vi "BusB FINS initialization Packet Encode.vi"(8 "error in":errorcluster, 11 "BusB Initialization Parameters":T1) -> (0 "error out":errorcluster, 2 "FCC Navigation send byte Array":u8[](array[numeric]) format="%x", 3 "BusB Initialization Parameters out":T1)   [LabVIEW 2016, in "Impedance Data Acquisition and Decoding.lvlib"]
uses:
  Impedance Data Acquisition and Decoding.lvlib
  BusB Initialization Parameters.ctl
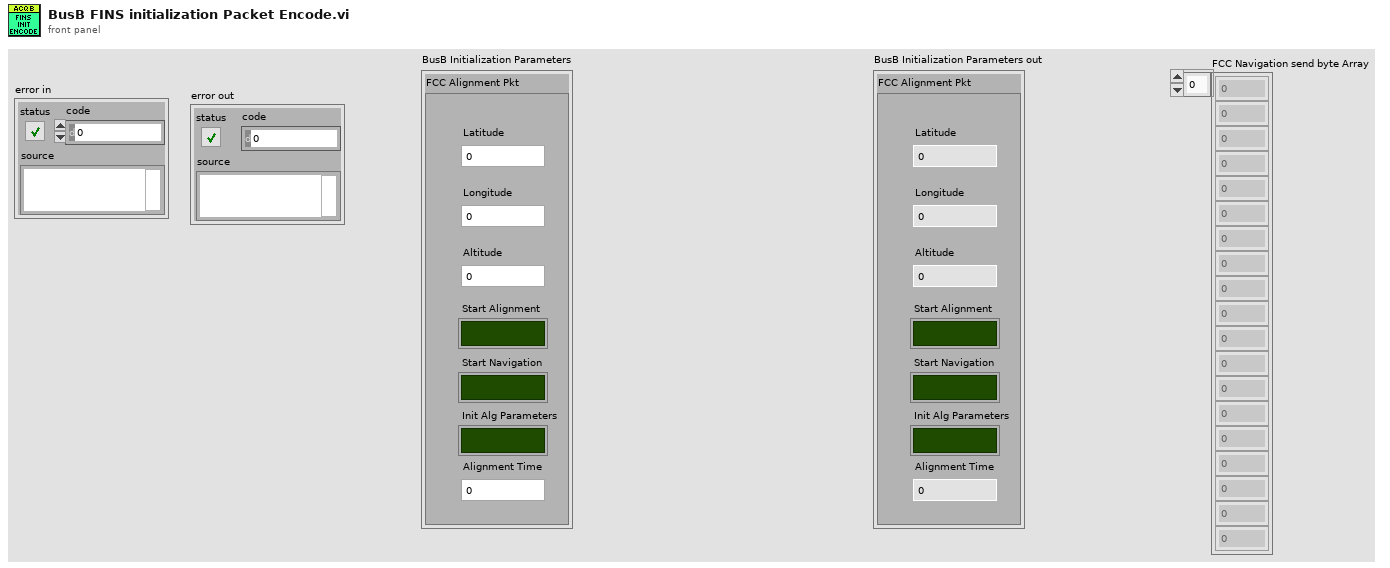
[diagram p1: front panel]
types:
  T1 = typedef "Impedance Data Acquisition and Decoding.lvlib/BusB Initialization Parameters.ctl" = cluster{"FCC Alignment Pkt":cluster{"Latitude":dbl, "Longitude":dbl, "Altitude":dbl, "Start Alignment":bool, "Alignment Time":u8, "Start Navigation":bool, "Init Alg Parameters":bool}}
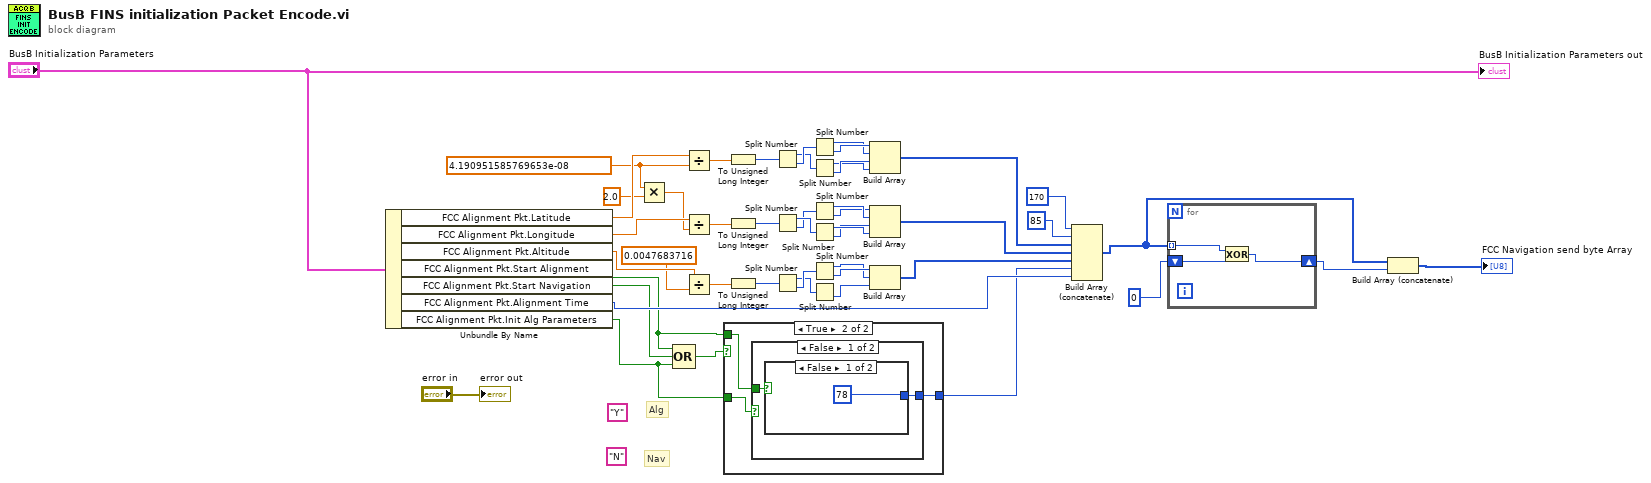
[diagram p0: block diagram]
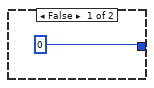
[diagram p2: hidden frame]
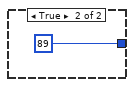
[diagram p3: hidden frame]
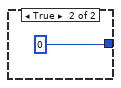
[diagram p4: hidden frame]
diagram:
  (unwired) "N"
  (unwired) "Y"
  w35 = 4.190951585769653e-08
  # "Nav"
  # "Alg"
  n1 = Unbundle By Name("BusB Initialization Parameters") -> ("FCC Alignment Pkt.Latitude"=w46:dbl, "FCC Alignment Pkt.Longitude"=w26:dbl, "FCC Alignment Pkt.Altitude"=w16:dbl, "FCC Alignment Pkt.Start Alignment"=w5:bool, "FCC Alignment Pkt.Start Navigation"=w7:bool, "FCC Alignment Pkt.Alignment Time"=w8:u8, "FCC Alignment Pkt.Init Alg Parameters"=w3:bool)
  n2 = Multiply(x=w35, y=2.0) -> (x*y=w25:dbl)
  n3 = Compound Arithmetic op=OR(w5, w7, w3) -> (w6:bool)
  n4 = Divide(x=w46, y=w35) -> (x/y=w45:dbl)
  n5 = Divide(x=w26, y=w25) -> (x/y=w27:dbl)
  n6 = Divide(x=w16, y=0.0047683716) -> (x/y=w23:dbl)
  n7 = case shown="True" w6 {
    tunnel: w5 -> [_ w51]
    tunnel: [u8 0 w50] -> w4
    tunnel: w3 -> [_ w49]
    frame False {
    }
    frame True {
      n8 = case shown="False" w49 {
        tunnel: w51 -> [w53 _]
        tunnel: [w52 u8 0] -> w50
        frame False {
          n9 = case shown="False" w53 {
            tunnel: [u8 78 u8 89] -> w52
            frame False {
            }
            frame True {
            }
          }
        }
        frame True {
        }
      }
    }
  }
  n10 = To Unsigned Long Integer(number=w45) -> (unsigned 32bit integer=w44:u32)
  n11 = To Unsigned Long Integer(number=w27) -> (unsigned 32bit integer=w28:u32)
  n12 = To Unsigned Long Integer(number=w23) -> (unsigned 32bit integer=w22:u32)
  n13 = Split Number(x=w44) -> (hi(x)=w42:u16, lo(x)=w43:u16)
  n14 = Split Number(x=w28) -> (hi(x)=w30:u16, lo(x)=w29:u16)
  n15 = Split Number(x=w22) -> (hi(x)=w20:u16, lo(x)=w21:u16)
  n16 = Split Number(x=w43) -> (hi(x)=w40:u8, lo(x)=w41:u8)
  n17 = Split Number(x=w42) -> (hi(x)=w38:u8, lo(x)=w39:u8)
  n18 = Split Number(x=w29) -> (hi(x)=w32:u8, lo(x)=w31:u8)
  n19 = Split Number(x=w30) -> (hi(x)=w34:u8, lo(x)=w33:u8)
  n20 = Split Number(x=w21) -> (hi(x)=w18:u8, lo(x)=w19:u8)
  n21 = Split Number(x=w20) -> (lo(x)=w17:u8)  [unwired: 1 out]
  n22 = Build Array(w41, w40, w39, w38) -> (w37:u8[])
  n23 = Build Array(w31, w32, w33, w34) -> (w24:u8[])
  n24 = Build Array(w19, w18, w17) -> (w14:u8[])
  n25 = Build Array (concatenate)(u8 170, u8 85, w37, w24, w14, w4, w8) -> (w10:u8[])
  n26 = for {
    tunnel: w10 -> [w59] mode=indexing
    shift-right: [w57] -> w2
    shift-left: u8 0 -> [w58]
    n27 = Exclusive Or(1:w58, 2:w59) -> (0:w57:u8)
  }
  n28 = Build Array (concatenate)(w10, w2) -> (→"FCC Navigation send byte Array":u8[])
  "error out" <- "error in"
  "BusB Initialization Parameters out" <- "BusB Initialization Parameters"
